vi "TTA_Update_Test_Status_Global.vi"(8 "error in":errorcluster, 11 "Test Status":string) -> (0 "error out":errorcluster)   [LabVIEW 2016]
uses:
  TTA_Globals/Test_Status.vi
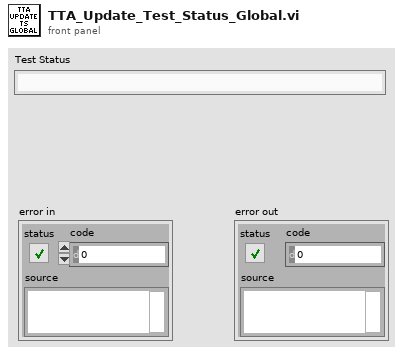
[diagram p1: front panel]
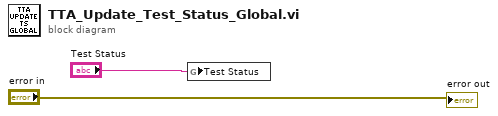
[diagram p0: block diagram]
diagram:
  n1 = global write "Test_Status.vi" "Test Status"("Test Status") -> ()
  "error out" <- "error in"
